vi "Untitled 4.vi"() -> ()   [LabVIEW 2019]
uses:
  <vilib>/userdefined/High Color/IMAQdx.ctl
  <vilib>/vision/driver/NI_Vision_Acquisition_Software.lvlib
  <resource>/objmgr/imaqdx.rc
panel:
  out "Processed Frames per Second":dbl
  out "Acquired Frames per Second":dbl
  out "error out":errorcluster
  out "Image":T1(plugin-control)
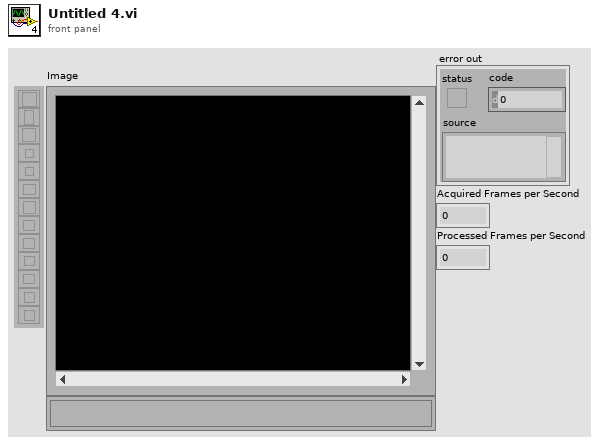
[diagram p1: front panel]
types:
  T1 = typedef "IMAQ Image.ctl" = refnum<image>
  T2 = typedef "Image Type" = u32
  T3 = typedef "IMAQdx.ctl" = refnum<k21>
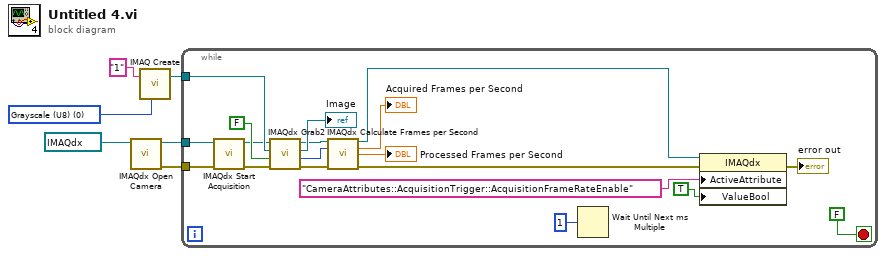
[diagram p0: block diagram]
diagram:
  w3 = T2 0 items=["Grayscale (U8)", "Grayscale (I16)", "Grayscale (SGL)", "Complex (CSG)", "RGB (U32)", "HSL (U32)", "RGB (U64)", "Grayscale (U16)"] ("Image Type")
  n1 = call <vilib>:"IMAQdx Open Camera.vi"("Session In"=T3 "cam5") -> ("error out"=w2:errorcluster, "Session Out"=w1:T3)  [unwired: 9 in]
  n2 = call "IMAQ Create"("Image Name"="1", "Image Type"=w3) -> ("New Image"=w5:T1)  [unwired: 3 in, 1 out]
  n3 = while {
    tunnel: w5 -> [w23]
    tunnel: w2 -> [w21]
    tunnel: w1 -> [w20]
    stop <- FALSE stop-if-true
    n4 = call <vilib>:"IMAQdx Start Acquisition.vi"("error in"=w21, "Session In"=w20) -> ("error out"=w19:errorcluster, "Session Out"=w18:T3)  [unwired: 8 in]
    n5 = call <vilib>:"IMAQdx Grab2.vi"("error in"=w19, "Wait for Next Buffer? (Yes)"=FALSE, "Image In"=w23, "Session In"=w18) -> ("error out"=w14:errorcluster, "Buffer Number Out"=w15:u32, "Image Out"=→"Image":T1, "Session Out"=w16:T3)  [unwired: 4 in]
    n6 = call <vilib>:"IMAQdx Calculate Frames per Second.vi"("Session In"=w16, "Buffer Number"=w15, "error in (no error)"=w14) -> ("Session Out"=w11:T3, "Acquired Frames per Second"=→"Acquired Frames per Second":dbl, "Processed Frames per Second"=→"Processed Frames per Second":dbl, "error out"=w10:errorcluster)  [unwired: 6 in, 3 out]
    n7 = Wait Until Next ms Multiple(millisecond multiple=u32 1) -> ()  [unwired: 1 out]
    n8 = property class="IMAQdx"(reference=w11, error in=w10, "ActiveAttribute"="CameraAttributes::AcquisitionTrigger::AcquisitionFrameRateEnable", "ValueBool"=TRUE) -> (error out=→"error out":errorcluster)  [unwired: 1 out]
  }
